vi "DB-DecodePageID.vi"(0 "PageID":string) -> (6 "Decoded Page ID":string)   [LabVIEW 2013]
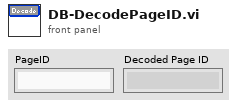
[diagram p1: front panel]
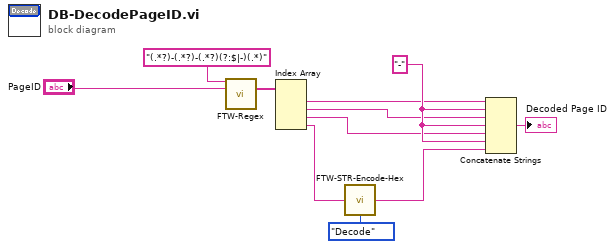
[diagram p0: block diagram]
diagram:
  w9 = "-" ("string")
  n1 = call "FTW-Regex.vi"("Regular Expression"="(.*?)-(.*?)-(.*?)(?:$|-)(.*)" ("regular expression"), "Input String"="PageID") -> ("Submatches"=w2:string[])  [unwired: 9 in, 4 out]
  n2 = Index Array(array=w2) -> (element #1=w6:string, element #2=w7:string, element #3=w8:string, element #4=w4:string)  [unwired: 4 in]
  n3 = call "FTW-STR-Encode-Hex.vi"("Input"=w4, "Direction"=enum16{"Encode", "Decode"}."Decode") -> ("Output"=w10:string)
  n4 = Concatenate Strings(w6, w9, w7, w9, w8, w9, w10) -> (→"Decoded Page ID":string)
